vi "Send Alternative Long Execution Method.vi"(7 "Message Priority (Normal)":T2=enum."Normal", 8 "error in (no error)":errorcluster, 10 "Async Call Method":T1, 11 "Message Enqueuer":refnum<class "Message Enqueuer.lvclass">) -> (0 "error out":errorcluster, 3 "Message Enqueuer out":refnum<class "Message Enqueuer.lvclass">)   [LabVIEW 2021, in "Async Methods Actor Example.lvlib" / "Alternative Long Execution Method Msg.lvclass"]
doc: "This VI sends the message to an actor."
uses:
  Alternative Long Execution Method Msg.lvclass
  <vilib>/ActorFramework/Message Enqueuer/Message Enqueuer.lvclass
  <vilib>/ActorFramework/Message Enqueuer/Message Priority.ctl
  Async Methods Actor/Async Methods Actor/Async Call Method.ctl
  C:/Projects/Async Methods Actor/Async Methods Actor/Async Methods Actor Messages/Async Message/Async Message.lvclass
  C:/Program Files/National Instruments/LabVIEW 2021/vi.lib/ActorFramework/Message/Message.lvclass
  Async Methods Actor/Async Methods Actor Messages/Async Message/Async Message.lvclass/Async Message.ctl
  <vilib>/ActorFramework/Message Enqueuer/Message Enqueuer.lvclass/Message Enqueuer.ctl
  Async Methods Actor/Async Methods Actor Messages/Async Message/Write Async Call Method.vi
  <vilib>/ActorFramework/Message Priority Queue/Priority Enqueue.vi
  Alternative Long Execution Method Msg.lvclass/Alternative Long Execution Method Msg.ctl
  Async Methods Actor/Async Methods Actor/Async Methods Actor.lvclass
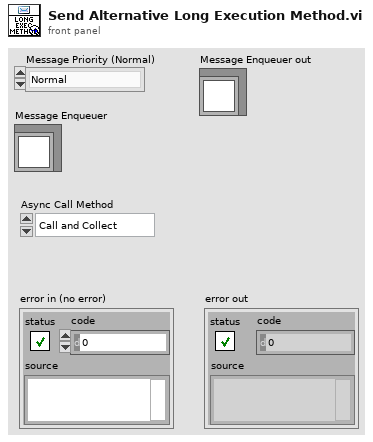
[diagram p1: front panel]
types:
  T1 = typedef "Async Methods Actor.lvlib/Async Methods Actor.lvclass/Async Call Method.ctl" = enum16{"Call and Collect", "Call and Forget"}
  T2 = typedef "Actor Framework.lvlib/Message Enqueuer.lvclass/Message Priority.ctl" = enum16{"Low", "Normal", "High"}
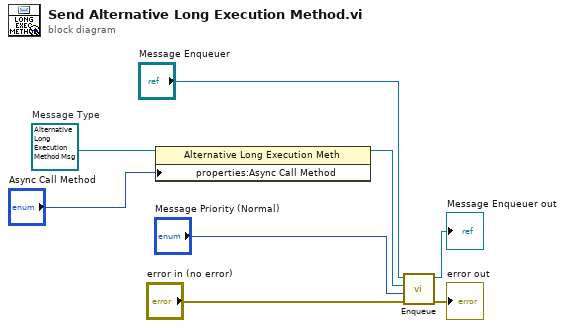
[diagram p0: block diagram]
diagram:
  w5 = refnum<class "Alternative Long Execution Method Msg.lvclass"> refnum  # Message Type
  n1 = property class="Alternative Long Execution Meth"(reference=w5, "properties:Async Call Method"="Async Call Method") -> (reference out=w2:refnum<class "Alternative Long Execution Method Msg.lvclass">)  [unwired: 1 in, 1 out]
  n2 = call <vilib>:"Enqueue.vi"("error in (no error)"="error in (no error)", "Message Priority (Normal)"="Message Priority (Normal)", "Message"=w2, "Message Enqueuer in"="Message Enqueuer") -> ("error out"=→"error out":errorcluster, "Message Enqueuer out"=→"Message Enqueuer out":refnum<class "Message Enqueuer.lvclass">)  [unwired: 6 in]
